vi "Initialize.vi"(8 "error in (no error)":errorcluster, 9 "Reset (F)":bool, 10 "IdQuery (F)":bool, 11 "IviFgen in":refnum<class "IviFgen.lvclass">) -> (0 "error out":errorcluster, 3 "IviFgen out":refnum<class "IviFgen.lvclass">)   [LabVIEW 2018, in "FgenPlugins.lvlib" / "IviFgen.lvclass"]
uses:
  IviFgen.lvclass
  X:/Projects/NistPluggableModules/dev/NistPluggableModules/FGen/FgenPlugins/FgenPluginBaseClass/FgenPluginsBase.lvclass
  FgenPluginBaseClass/FgenPluginsBase.lvclass/FgenPluginsBase.ctl
  FgenPluginBaseClass/Accessors/Read Channels.vi
  FgenPluginBaseClass/Accessors/Write Channels.vi
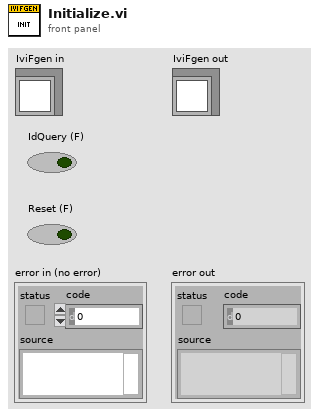
[diagram p1: front panel]
types:
  T1 = cluster{bool, "instrument handle out":refnum<k15>}[]
  T2 = typedef "Channel.ctl" = cluster{"Name":string, "Enabled":bool, "Operation":enum16{"Continuous", "Burst"}, "Impedance (50)":dbl, "Handle":string, "Connected":bool, "Mode (Function)":enum16{"Function", "Arbitrary", "Sequence"}}
  T3 = cluster{"f":bool, "instrument handle out":refnum<k15>}
  T4 = cluster{"f":bool, "instrument handle out":refnum<k15>}[]
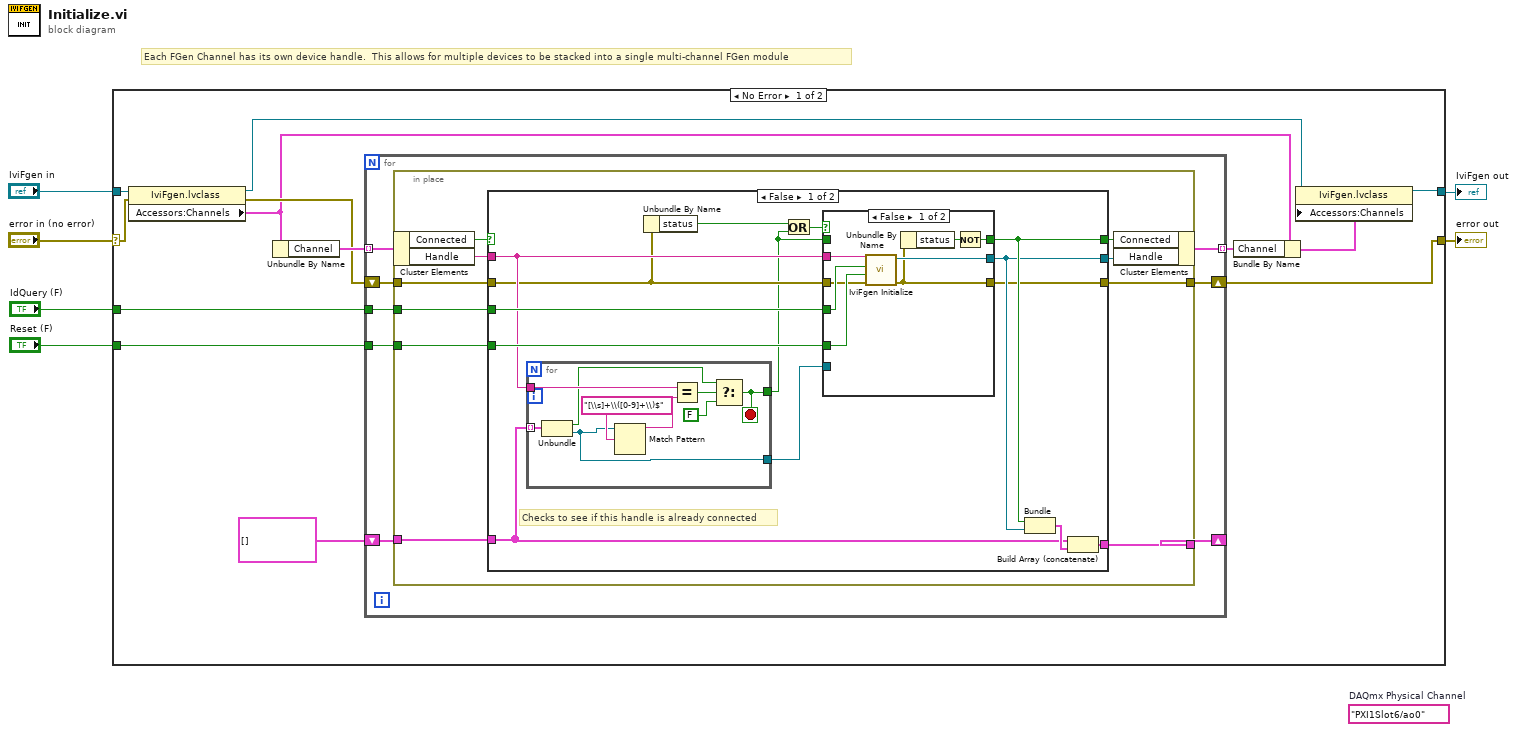
[diagram p0: block diagram]
diagram:
  (unwired) tag "PXI1Slot6/ao0"  # DAQmx Physical Channel
  # "Each FGen Channel has its own device handle.  This allows for multiple devices to be stacked into a single multi-channel FGen module"
  n1 = case shown="No Error" "error in (no error)" {
    selector: "error in (no error)" -> [w16 w76]
    tunnel: "IviFgen in" -> [w19 w77]
    tunnel: [w11 w77] -> w3
    tunnel: [w12 w76] -> w4
    tunnel: "IdQuery (F)" -> [w17 _]
    tunnel: "Reset (F)" -> [w14 _]
    frame No Error {
      n2 = property class="IviFgen.lvclass"(reference=w19, error in=w16) -> (reference out=w7:refnum<class "IviFgen.lvclass">, error out=w15:errorcluster, "Accessors:Channels"=w10:cluster{"Count":u16, "Channel":T2[]})
      n3 = Unbundle By Name(w10) -> ("Channel"=w18:T2[])
      n4 = for {
        tunnel: w18 -> [w27] mode=indexing
        tunnel: w17 -> [w26]
        tunnel: w14 -> [w25]
        shift-right: [w23] -> _
        shift-left: T1 [] -> [w22]
        shift-right: [w21] -> w12
        shift-left: w15 -> [w24]
        tunnel: [w20] -> w9 mode=indexing
        n5 = in-place {
          in-place-border: w26 -> [w37]
          in-place-border: w25 -> [w36]
          in-place-border: w24 -> [w29]
          in-place-border: [w33] -> w23
          in-place-border: w22 -> [w32]
          in-place-border: [w30] -> w21
          n6 = in-place-cluster #1(w27) -> ("Connected"=w28:bool, "Handle"=w31:string)
          n7 = case shown="False" w28 {
            selector: w28 -> [_ w75]
            tunnel: w37 -> [w51 _]
            tunnel: w36 -> [w50 _]
            tunnel: [w49 w75] -> w35
            tunnel: [w48 w74] -> w34
            tunnel: [w46 w72] -> w33
            tunnel: w32 -> [w45 w72]
            tunnel: w31 -> [w44 w74]
            tunnel: [w43 w73] -> w30
            tunnel: w29 -> [w42 w73]
            frame False {
              # "Checks to see if this handle is already connected"
              n8 = for {
                tunnel: w45 -> [w59] mode=indexing
                tunnel: w44 -> [w60]
                tunnel: [w57] -> w38
                tunnel: [w52] -> w41
                stop <- w57 stop-if-true
                n9 = Unbundle(w59) -> (w55:bool, "instrument handle out"=w52:refnum<k15>)
                n10 = Match Pattern(string=w52, regular expression="[\\s]+\\([0-9]+\\)$") -> (before substring=w54:string)  [unwired: 1 in, 3 out]
                n11 = Equal?(x=w60, y=w54) -> (x = y?=w58:bool)
                n12 = Select(t=w55, s=w58, f=FALSE) -> (s? t:f=w57:bool)
              }
              n13 = Unbundle By Name(w42) -> ("status"=w39:bool)
              n14 = Or(x=w39, y=w38) -> (x .or. y?=w40:bool)
              n15 = case shown="False" w40 {
                tunnel: [w62 w69] -> w49
                tunnel: w44 -> [w68 _]
                tunnel: [w67 w70] -> w48
                tunnel: w51 -> [w66 _]
                tunnel: w50 -> [w65 _]
                tunnel: w42 -> [w64 w71]
                tunnel: [w61 w71] -> w43
                tunnel: w41 -> [_ w70]
                tunnel: w38 -> [_ w69]
                frame False {
                  n16 = call <vilib>:"IviFgen Initialize.vi"("error in (no error)"=w64, "reset device (true)"=w65, "id query (true)"=w66, "logical name (\"SampleFGen\")"=w68) -> ("error out"=w61:errorcluster, "instrument handle out"=w67:refnum<k15>)  [unwired: 6 in]
                  n17 = Unbundle By Name(w61) -> ("status"=w63:bool)
                  n18 = Not(x=w63) -> (.not. x?=w62:bool)
                }
                frame True {
                }
              }
              n19 = Bundle("f"=w49, "instrument handle out"=w48) -> (w47:T3)  [unwired: 1 in]
              n20 = Build Array (concatenate)(w45, w47) -> (w46:T4)
            }
            frame True {
            }
          }
          n21 = in-place-cluster #1("Connected"=w35, "Handle"=w34) -> (w20:T2)
        }
      }
      n22 = Bundle By Name(cluster=w10, "Channel"=w9) -> (w8:cluster{"Count":u16, "Channel":T2[]})
      n23 = property class="IviFgen.lvclass"(reference=w7, "Accessors:Channels"=w8) -> (reference out=w11:refnum<class "IviFgen.lvclass">)  [unwired: 1 in, 1 out]
    }
    frame Error {
    }
  }
  "error out" <- w4
  "IviFgen out" <- w3
